vi "example_01_setup_path.vi"() -> ()   [LabVIEW 2015, in "lv-bin.lvlib" / "v1.lvlib"]
doc: "example_01_setup_path.vi is used to provide an example of how you can add one or more paths to a functional global that can be used to search for a file (identical to how pathing works for command shells)."
uses:
  v1.lvlib
  advanced/add_data_path_single.vi
panel:
  out "error out":errorcluster
  out "paths_after":path[](array[path])
  out "paths_before":path[](array[path])
  in  "path":path=path "" caption="start path"
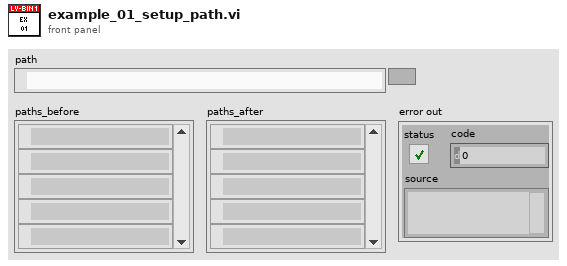
[diagram p1: front panel]
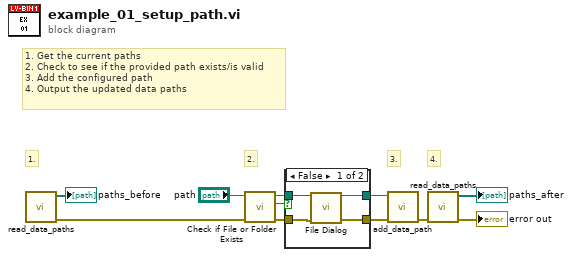
[diagram p0: block diagram]
diagram:
  # "1. Get the current paths\n2. Check to see if the provided path exists/is valid\n3. Add the configured path\n4. Output the updated data paths"
  # "4."
  # "3."
  # "2."
  # "1."
  n1 = call "read_data_paths.vi"() -> ("error out"=w5:errorcluster, "path [] out"=→"paths_before":path[])  [unwired: 10 in]
  n2 = call <vilib>:"Check if File or Folder Exists.vi"("error in (no error)"=w5, "path"="path") -> ("error out"=w6:errorcluster, "file or folder exists?"=w7:bool, "dup path"=w8:path)  [unwired: 7 in]
  n3 = case shown="False" w7 {
    tunnel: [w15 w16] -> w11
    tunnel: [w14 w17] -> w10
    tunnel: w8 -> [w13 w16]
    tunnel: w6 -> [w12 w17]
    frame False {
      n4 = call "File Dialog"("start path"=w13, "error in"=w12) -> ("selected path"=w15:path, "error out"=w14:errorcluster)  [unwired: 10 in, 2 out]
    }
    frame True {
    }
  }
  n5 = call-poly "add_data_path.vi"("error in (no error)"=w10, "path_to_add"=w11) -> ("error out"=w3:errorcluster)  [unwired: 9 in]
  n6 = call "read_data_paths.vi"("error in (no error)"=w3) -> ("error out"=→"error out":errorcluster, "path [] out"=→"paths_after":path[])  [unwired: 9 in]
